vi "质控启动器.vi"(8 "error in (no error)":errorcluster, 9 "加标体积":sgl, 10 "流程控制":T1, 11 "Slave ID":T2) -> (0 "error out":errorcluster)   [LabVIEW 2016, in "质控单元V2.lvlib"]
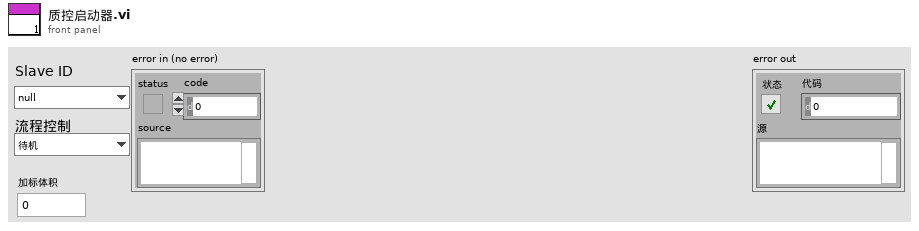
[diagram p1: front panel]
types:
  T1 = typedef "质控单元V2.lvlib/质控标准流程.ctl" = enum16{"待机", "启动进样流程", "启动加标流程", "启动排液流程", "启动水样润洗流程", "启动加标润洗流程", "停止流程", "启动搅拌流程", "停止搅拌流程"}
  T2 = typedef "质控单元V2.lvlib/质控slave id.ctl" = enum16{"null", "氨氮", "总磷", "总氮", "CODMn", "CODCr"}
  T3 = typedef "质控单元V2.lvlib/质控流程控制.ctl" = enum16{"待机", "启动进样流程", "启动加标流程", "启动排液流程", "停止流程", "加标（单独一步骤）"}
  T4 = typedef "质控单元V2.lvlib/质控组合命令区.ctl" = enum16{"停止", "进水样", "排废液", "进空气（搅拌）", "定量（反转定量）", "加标"}
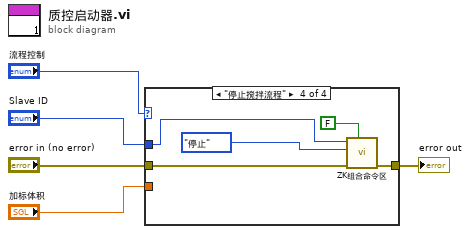
[diagram p0: block diagram]
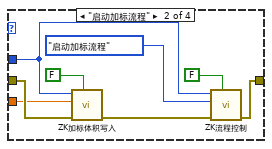
[diagram p3: hidden frame]
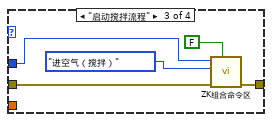
[diagram p4: hidden frame]
diagram:
  n1 = case shown="\"停止搅拌流程\"" "流程控制" {
    tunnel: "Slave ID" -> [_ w9 w19 w24]
    tunnel: [w6 w10 w16 w21] -> w1
    tunnel: "error in (no error)" -> [w6 w13 w17 w22]
    tunnel: "加标体积" -> [_ w12 _ _]
    frame "待机", Default {
    }
    frame "启动加标流程" {
      n2 = call "ZK加标体积写入.vi"("是否启用通讯通知"=FALSE, "error in (no error)"=w13, "加标体积"=w12, "Slave ID"=w9) -> ("error out"=w11:errorcluster)  [unwired: 7 in]
      n3 = call "ZK流程控制.vi"("是否启用通讯通知"=FALSE, "error in (no error)"=w11, "流程控制"=质控流程控制."启动加标流程", "Slave ID"=w9) -> ("error out"=w10:errorcluster)  [unwired: 7 in]
    }
    frame "启动搅拌流程" {
      n4 = call "ZK组合命令区.vi"("是否启用通讯通知"=FALSE, "error in (no error)"=w17, "组合命令区"=质控组合命令区."进空气（搅拌）", "Slave ID"=w19) -> ("error out"=w16:errorcluster)  [unwired: 7 in]
    }
    frame "停止搅拌流程" {
      n5 = call "ZK组合命令区.vi"("是否启用通讯通知"=FALSE, "error in (no error)"=w22, "组合命令区"=质控组合命令区."停止", "Slave ID"=w24) -> ("error out"=w21:errorcluster)  [unwired: 7 in]
    }
  }
  "error out" <- w1
